vi "from string array.vi"(8 "error in (no error)":errorcluster, 9 "String Array":string[][](array[string]), 10 "version":string, 11 "PID Module 2 configuration in":refnum<class "PID Module 2 configuration.lvclass">) -> (0 "error out":errorcluster, 3 "PID Module 2 configuration out":refnum<class "PID Module 2 configuration.lvclass">)   [LabVIEW 2015, in "PID Module 2 configuration.lvclass"]
uses:
  PID Module 2 configuration.lvclass
  PID Module 2 configuration.lvclass/PID Module 2 configuration.ctl
  Write Lines.vi
  Get Line Name.vi
  <vilib>/NI/Tag Bus Module Framework/module configuration/FindDuplicate.vi
  <vilib>/Utility/error.llb/Error Cluster From Error Code.vi
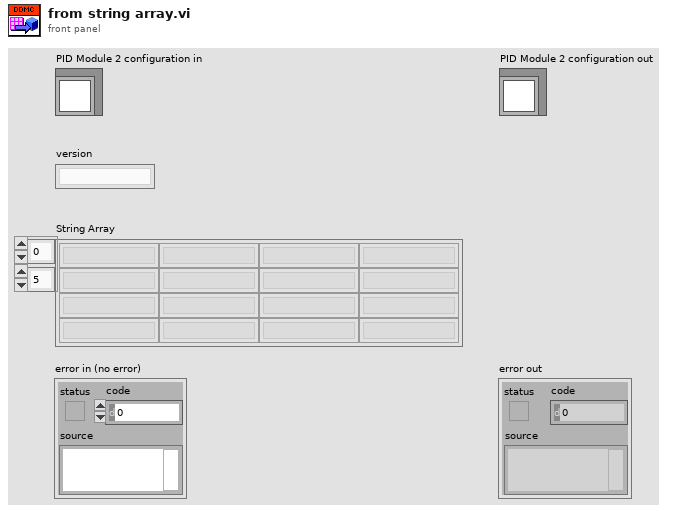
[diagram p1: front panel]
types:
  T1 = typedef "PID Module 2 configuration.lvclass/Line.ctl" = cluster{"PID ID":string, "Setpoint":refnum<class "TBM channel.lvclass">, "Variable":refnum<class "TBM channel.lvclass">, "Output":refnum<class "TBM channel.lvclass">, "Output High":refnum<class "TBM channel.lvclass">, "Output Low":refnum<class "TBM channel.lvclass">, "P":refnum<class "TBM channel.lvclass">, "I":refnum<class "TBM channel.lvclass">, "D":refnum<class "TBM channel.lvclass">}
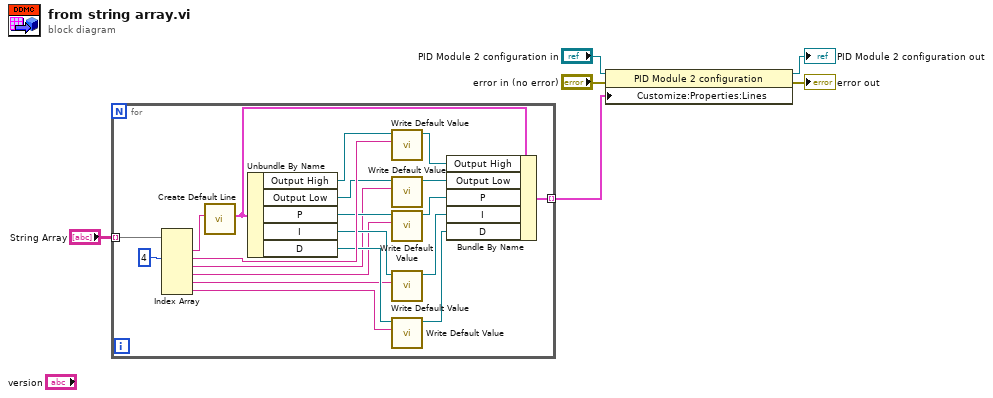
[diagram p0: block diagram]
diagram:
  n1 = for {
    tunnel: "String Array" -> [w26] mode=indexing
    tunnel: [w25] -> w1 mode=indexing
    n2 = Index Array(array=w26, index #2=4 ("index")) -> (element #1=w24:string, element #2=w20:string, element #3=w10:string, element #4=w9:string, element #5=w8:string, element #6=w7:string)  [unwired: 5 in]
    n3 = call "Create Default Line.vi"("Line Name"=w24) -> ("Default Line"=w23:T1)  [unwired: 10 in]
    n4 = Unbundle By Name(w23) -> ("Output High"=w21:refnum<class "TBM channel.lvclass">, "Output Low"=w16:refnum<class "TBM channel.lvclass">, "P"=w17:refnum<class "TBM channel.lvclass">, "I"=w18:refnum<class "TBM channel.lvclass">, "D"=w19:refnum<class "TBM channel.lvclass">)
    n5 = call "Write Default Value.vi"("Data"=w20, "Channel in"=w21) -> ("Channel out"=w22:refnum<class "TBM channel.lvclass">)  [unwired: 9 in]
    n6 = call "Write Default Value.vi"("Data"=w10, "Channel in"=w16) -> ("Channel out"=w15:refnum<class "TBM channel.lvclass">)  [unwired: 9 in]
    n7 = call "Write Default Value.vi"("Data"=w9, "Channel in"=w17) -> ("Channel out"=w14:refnum<class "TBM channel.lvclass">)  [unwired: 9 in]
    n8 = call "Write Default Value.vi"("Data"=w8, "Channel in"=w18) -> ("Channel out"=w13:refnum<class "TBM channel.lvclass">)  [unwired: 9 in]
    n9 = call "Write Default Value.vi"("Data"=w7, "Channel in"=w19) -> ("Channel out"=w12:refnum<class "TBM channel.lvclass">)  [unwired: 9 in]
    n10 = Bundle By Name(cluster=w23, "Output High"=w22, "Output Low"=w15, "P"=w14, "I"=w13, "D"=w12) -> (w25:T1)
  }
  n11 = property class="PID Module 2 configuration"(reference="PID Module 2 configuration in", error in="error in (no error)", "Customize:Properties:Lines"=w1) -> (reference out=→"PID Module 2 configuration out":refnum<class "PID Module 2 configuration.lvclass">, error out=→"error out":errorcluster)
